vi "Generate Piece.vi"() -> (3 "Piece":T1)   [LabVIEW 2017, in "Game Engine.lvlib" / "Game Engine.lvclass"]
uses:
  Game Engine.lvclass
  Piece.ctl
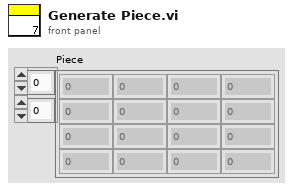
[diagram p1: front panel]
types:
  T1 = typedef "Game Engine.lvlib/Game Engine.lvclass/Piece.ctl" = u32[][]
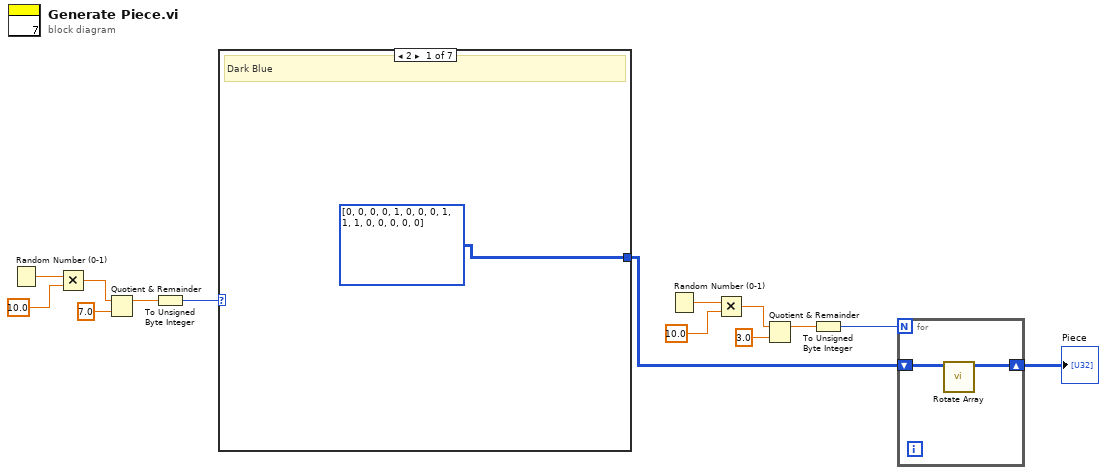
[diagram p0: block diagram]
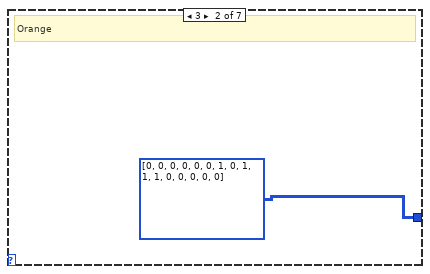
[diagram p2: hidden frame]
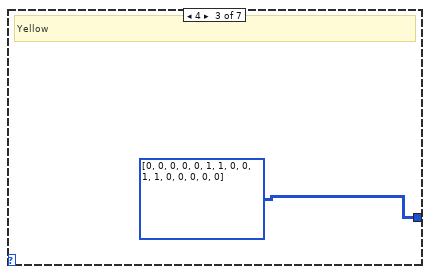
[diagram p3: hidden frame]
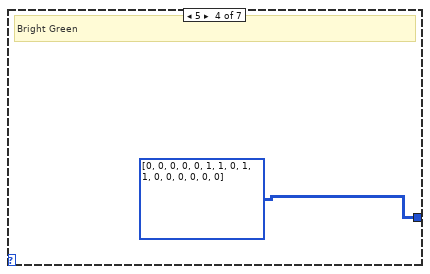
[diagram p4: hidden frame]
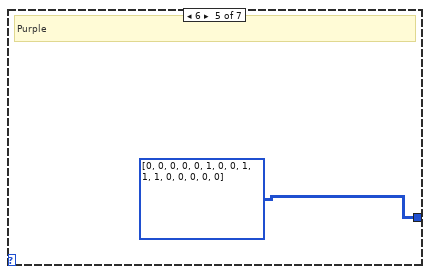
[diagram p5: hidden frame]
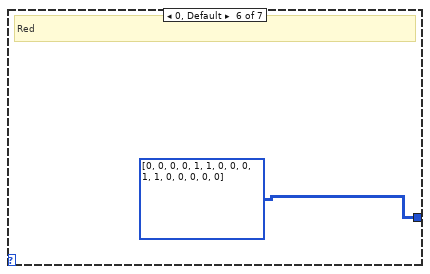
[diagram p6: hidden frame]
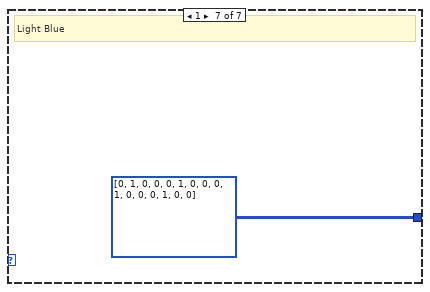
[diagram p7: hidden frame]
diagram:
  n1 = Random Number (0-1)() -> (number: 0 to 1=w14:dbl)
  n2 = Multiply(x=w14, y=10.0) -> (x*y=w12:dbl)
  n3 = Quotient & Remainder(x=w12, y=7.0) -> (x-y*floor(x/y)=w9:dbl)  [unwired: 1 out]
  n4 = To Unsigned Byte Integer(number=w9) -> (unsigned 8bit integer=w10:u8)
  n5 = case shown="2" w10 {
    tunnel: [T1 [[0, 0, 0, 0], [1, 0, 0, 0], [1, 1, 1, 0], [0, 0, 0, 0]] ("Piece") T1 [[0, 0, 0, 0], [0, 0, 1, 0], [1, 1, 1, 0], [0, 0, 0, 0]] ("Piece") T1 [[0, 0, 0, 0], [0, 1, 1, 0], [0, 1, 1, 0], [0, 0, 0, 0]] ("Piece") T1 [[0, 0, 0, 0], [0, 1, 1, 0], [1, 1, 0, 0], [0, 0, 0, 0]] ("Piece") T1 [[0, 0, 0, 0], [0, 1, 0, 0], [1, 1, 1, 0], [0, 0, 0, 0]] ("Piece") T1 [[0, 0, 0, 0], [1, 1, 0, 0], [0, 1, 1, 0], [0, 0, 0, 0]] ("Piece") T1 [[0, 1, 0, 0], [0, 1, 0, 0], [0, 1, 0, 0], [0, 1, 0, 0]] ("Piece")] -> w2
    frame 2 {
      # "Dark Blue"
    }
    frame 3 {
      # "Orange"
    }
    frame 4 {
      # "Yellow"
    }
    frame 5 {
      # "Bright Green"
    }
    frame 6 {
      # "Purple"
    }
    frame 0, Default {
      # "Red"
    }
    frame 1 {
      # "Light Blue"
    }
  }
  n6 = Random Number (0-1)() -> (number: 0 to 1=w8:dbl)
  n7 = Multiply(x=w8, y=10.0) -> (x*y=w6:dbl)
  n8 = Quotient & Remainder(x=w6, y=3.0) -> (x-y*floor(x/y)=w4:dbl)  [unwired: 1 out]
  n9 = To Unsigned Byte Integer(number=w4) -> (unsigned 8bit integer=w3:u8)
  n10 = for {
    N: w3 -> [_]
    shift-right: [w22] -> w1
    shift-left: w2 -> [w23]
    n11 = call "Rotate Array.vi"("Array in"=w23) -> ("Array out"=w22:u32[][])  [unwired: 10 in]
  }
  "Piece" <- w1
